vi "GetWaveforms.vi"(1 "targetRef":refnum<k24>, 3 "error in":errorcluster) -> (8 "Waveforms":cluster{"Name":string, "ID":u64}[](array[cluster]), 10 "error out":errorcluster)   [LabVIEW 2014, in "Waveform-Processing-Custom-Device System Explorer.lvlib"]
uses:
  Waveform-Processing-Custom-Device System Explorer.lvlib
  NationalInstruments.VeriStand.SystemStorage
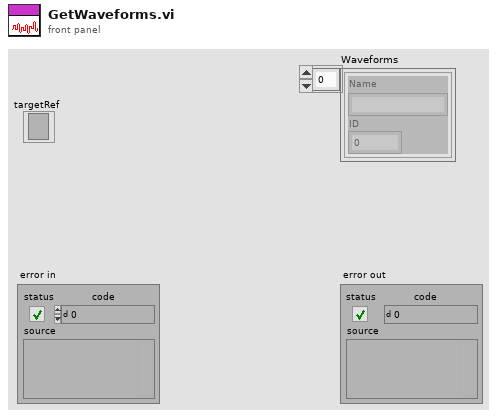
[diagram p1: front panel]
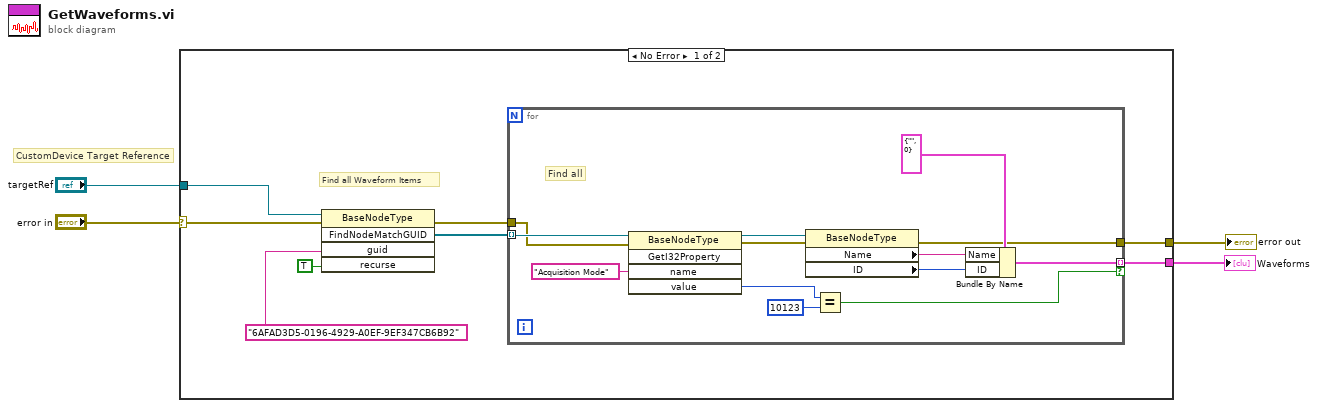
[diagram p0: block diagram]
diagram:
  # "CustomDevice Target Reference"
  n1 = case shown="No Error" "error in" {
    selector: "error in" -> [w12 w26]
    tunnel: [w5 w26] -> w3
    tunnel: "targetRef" -> [w11 _]
    tunnel: [w6 _] -> w1
    frame No Error {
      # "Find all Waveform Items"
      n2 = invoke class="BaseNodeType" method="FindNodeMatchGUID"(reference=w11, error in=w12, "guid"="6AFAD3D5-0196-4929-A0EF-9EF347CB6B92", "recurse"=TRUE) -> (error out=w7:errorcluster, "FindNodeMatchGUID"=w8:refnum<k24>[])  [unwired: 1 in, 3 out]
      n3 = for {
        tunnel: w8 -> [w25] mode=indexing
        tunnel: w7 -> [w20]
        tunnel: [w15] -> w6 mode=indexing if=w14
        tunnel: [w13] -> w5
        # "Find all"
        n4 = invoke class="BaseNodeType" method="GetI32Property"(reference=w25, error in=w20, "name"="Acquisition Mode") -> (reference out=w23:refnum<k24>, error out=w21:errorcluster, "value"=w17:i32)  [unwired: 2 in, 2 out]
        n5 = property class="BaseNodeType"(reference=w23, error in=w21) -> (error out=w13:errorcluster, "Name"=w22:string, "ID"=w18:u64)  [unwired: 1 out]
        n6 = Equal?(x=w17, y=10123) -> (x = y?=w14:bool)
        n7 = Bundle By Name(cluster=cluster{"Name":string, "ID":u64} {"Name"="", "ID"=0} ("Waveform"), "Name"=w22, "ID"=w18) -> (w15:cluster{"Name":string, "ID":u64})
      }
    }
    frame Error {
    }
  }
  "error out" <- w3
  "Waveforms" <- w1
